vi "HRM-Stage4-filter_waveform.vi"(8 "error in (no error)":errorcluster, 11 "Process data":T1={"Samples size (10)"=10, "Addition signal to remove"=0.0, "Unfiltered wf"={"t0"=timestamp(0 s since 1904-01-01), "dt"=1.0, "Y"=[]}, "Filtered wf"={"t0"=timestamp(0 s since 1904-01-01), "dt"=1.0, "Y"=[]}, "Heart Rate"=0.0, "Peak detect settings"={"Manual?"=FALSE, "Top"=0.0, "Bot"=0.0}, "User Events"={"Signal to remove"=refnum, "Sample size"=refnum, "Filtered wf"=refnum, "Unfiltered wf"=refnum, "Raw wf"=refnum, "Pulse"=refnum, "Stop"=refnum, "Feedback"=refnum, "Run Aqn?"=refnum, "Clear"=refnum, "Peak Det. Set."=refnum}}) -> (0 "error out":errorcluster, 3 "Process data out":T1={"Samples size (10)"=10, "Addition signal to remove"=0.0, "Unfiltered wf"={"t0"=timestamp(0 s since 1904-01-01), "dt"=1.0, "Y"=[]}, "Filtered wf"={"t0"=timestamp(0 s since 1904-01-01), "dt"=1.0, "Y"=[]}, "Heart Rate"=0.0, "Peak detect settings"={"Manual?"=FALSE, "Top"=0.0, "Bot"=0.0}, "User Events"={"Signal to remove"=refnum, "Sample size"=refnum, "Filtered wf"=refnum, "Unfiltered wf"=refnum, "Raw wf"=refnum, "Pulse"=refnum, "Stop"=refnum, "Feedback"=refnum, "Run Aqn?"=refnum, "Clear"=refnum, "Peak Det. Set."=refnum}})   [LabVIEW 2020]
uses:
  HRM-process-loop_cluster.ctl
  HRM-process-peak_detect_setting.ctl
  initclose/HRM-Stage4-User_events.ctl
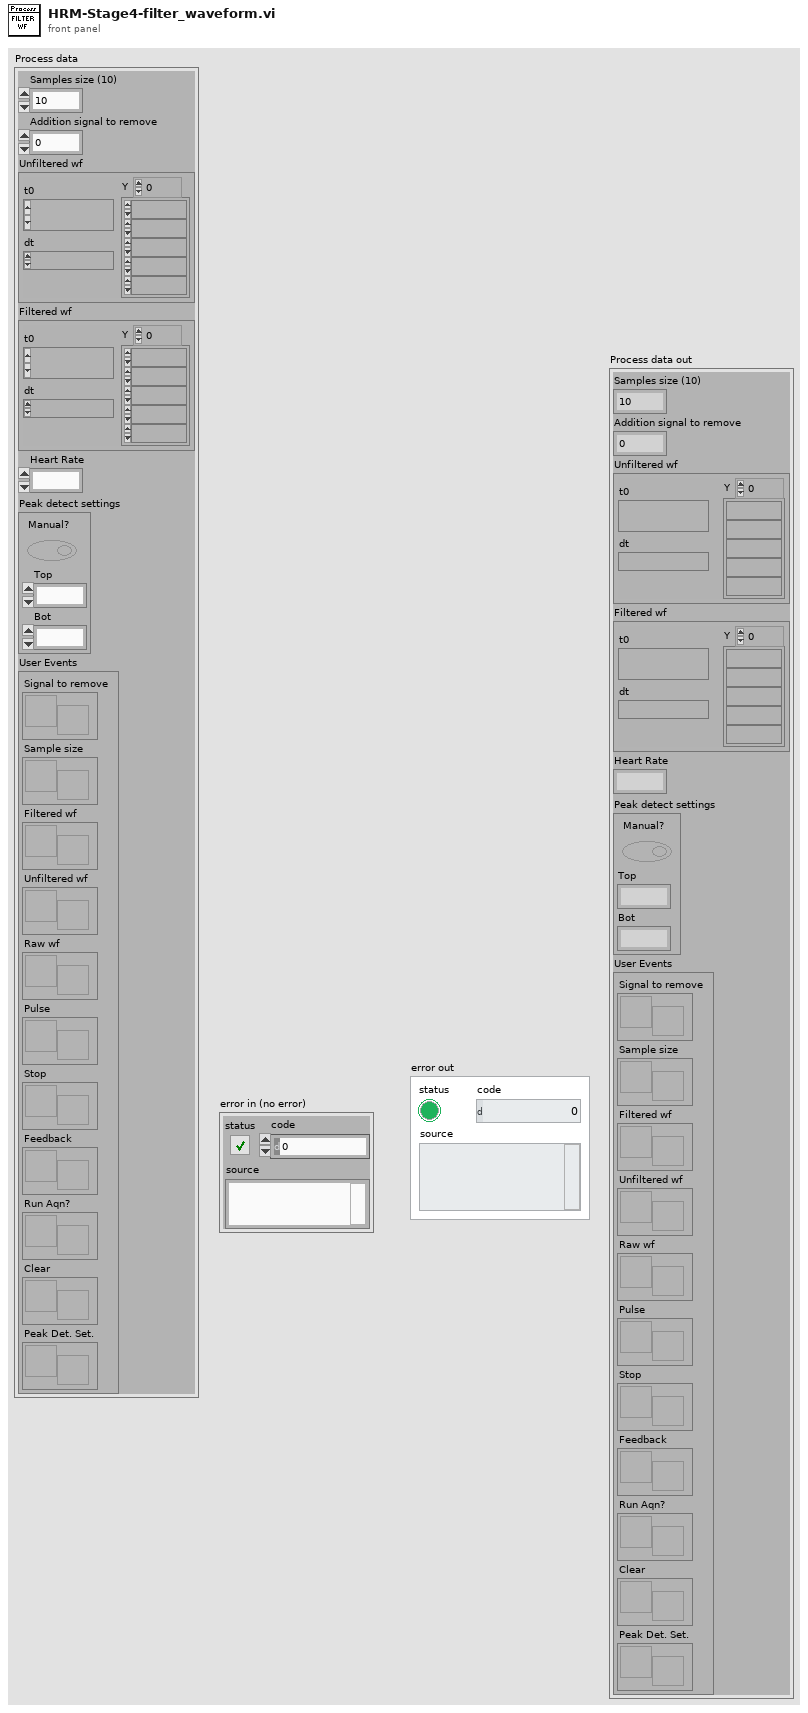
[diagram p1: front panel]
types:
  T1 = typedef "HRM-process-loop_cluster.ctl" = cluster{"Samples size (10)":i32, "Addition signal to remove":dbl, "Unfiltered wf":waveform(dbl), "Filtered wf":waveform(dbl), "Heart Rate":dbl, "Peak detect settings":T2, "User Events":T3}
  T2 = typedef "HRM-process-peak_detect_setting.ctl" = cluster{"Manual?":bool, "Top":dbl, "Bot":dbl}
  T3 = typedef "HRM-Stage4-User_events.ctl" = cluster{"Signal to remove":refnum<user-event>, "Sample size":refnum<user-event>, "Filtered wf":refnum<user-event>, "Unfiltered wf":refnum<user-event>, "Raw wf":refnum<user-event>, "Pulse":refnum<user-event>, "Stop":refnum<user-event>, "Feedback":refnum<user-event>, "Run Aqn?":refnum<user-event>, "Clear":refnum<user-event>, "Peak Det. Set.":refnum<user-event>}
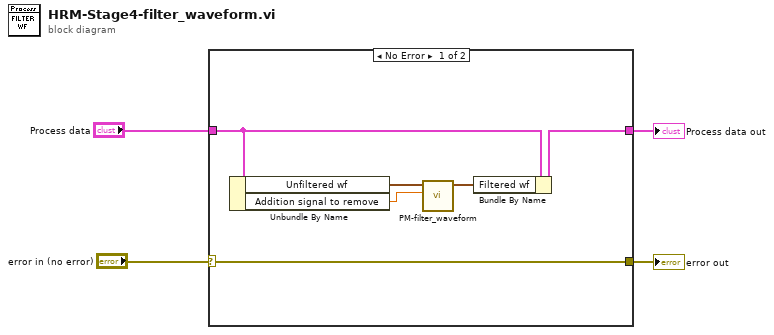
[diagram p0: block diagram]
diagram:
  n1 = case shown="No Error" "error in (no error)" {
    selector: "error in (no error)" -> [w10 w12]
    tunnel: [w10 w12] -> w3
    tunnel: "Process data" -> [w9 w11]
    tunnel: [w6 w11] -> w1
    frame No Error {
      n2 = Unbundle By Name(w9) -> ("Unfiltered wf"=w8:waveform(dbl), "Addition signal to remove"=w7:dbl)
      n3 = call "PM-filter_waveform.vi"("Addition signal to remove (0) [s]"=w7, "waveform in"=w8) -> ("waveform out"=w5:waveform(dbl))  [unwired: 8 in, 1 out]
      n4 = Bundle By Name(cluster=w9, "Filtered wf"=w5) -> (w6:T1)
    }
    frame Error {
    }
  }
  "Process data out" <- w1
  "error out" <- w3
